vi "Task Messung.vi"(3 "Gauge":refnum<vi>, 5 "Chart":refnum<vi>, 6 "Average":refnum<vi>, 7 "Graph":refnum<vi>, 11 "Channel in":T1) -> (0 "error out":errorcluster)   [LabVIEW 2018]
uses:
  <extravilib>/ChannelInstances/Tag-t'States Worker.ctl'/))Channel.ctl
  Type Definitions/States Worker.ctl
  <vilib>/DAQmx/read.llb/DAQmx Read (Analog Wfm 1Chan NSamp).vi
  <extravilib>/ChannelInstances/Tag-t'States Worker.ctl'/Read With Abort.vi
  <extravilib>/ChannelInstances/Tag-t'States Worker.ctl'/EndpointRead.vi
  <vilib>/DAQmx/miscellaneous.llb/DAQmx Fill In Error Info.vi
  <vilib>/Waveform/WDTOps.llb/WDT Append Waveforms DBL.vi
  <extravilib>/ChannelInstances/Tag-t'States Worker.ctl'.lvlib
panel:
  out "Number of Scans":i32
  # "Worker Task"
  # "Tasks:\n1) Messen\n2) Auswerten\n3) Pausieren"
  # "Communication:\nTag Channel"
  # "These tasks run in parallel\nto other loops!"
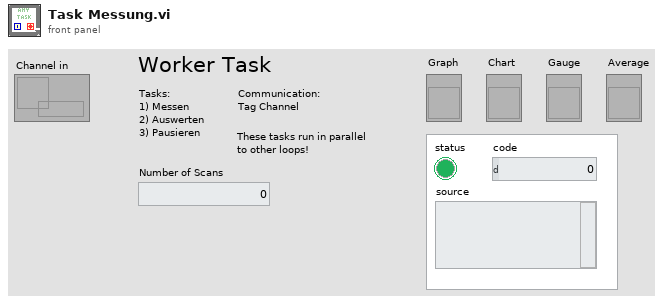
[diagram p1: front panel]
types:
  T1 = typedef "Tag-t'States Worker.ctl'.lvlib/))Channel.ctl" = refnum<queue>
  T2 = typedef "States Worker.ctl" = enum16{"Messen", "Pausieren", "Exit"}
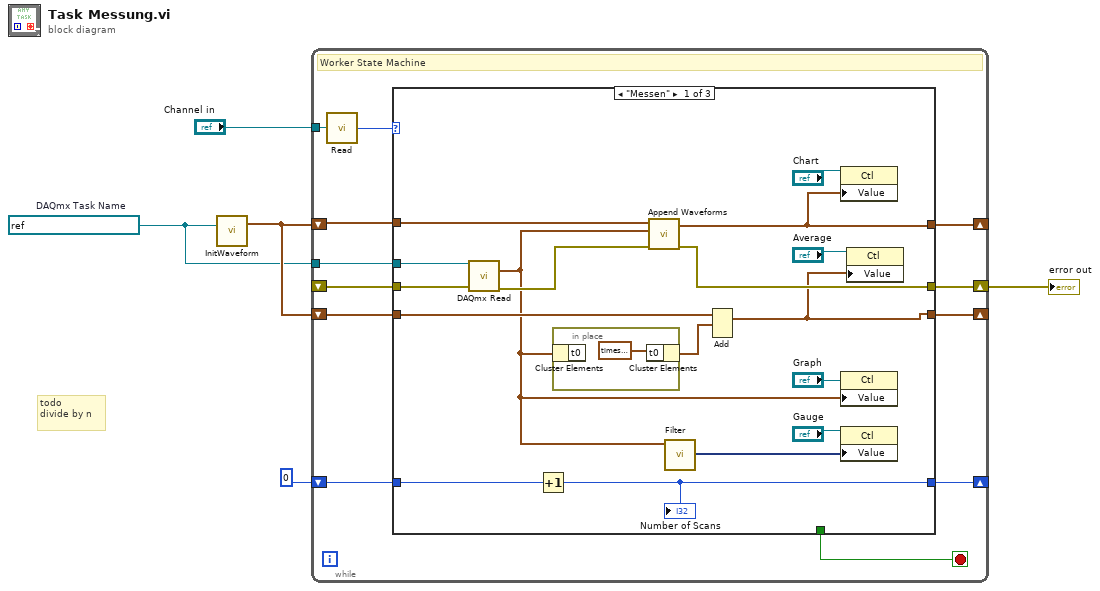
[diagram p0: block diagram]
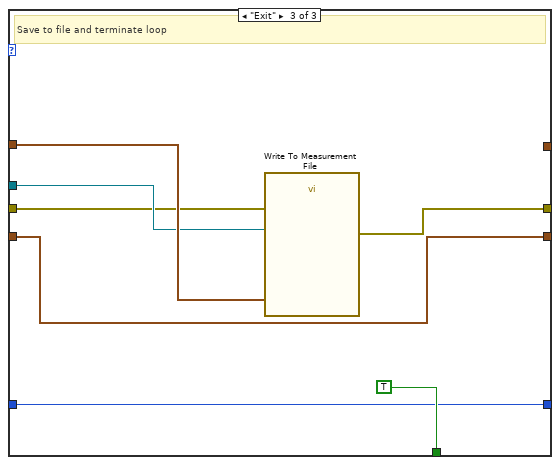
[diagram p3: hidden frame]
diagram:
  w2 = refnum<k21> "Spannung_1kHz100"  # DAQmx Task Name
  # "todo\ndivide by n"
  n1 = call "InitWaveform.vi"("Refnum in"=w2) -> ("Waveform"=w3:waveform(dbl))  [unwired: 10 in]
  n2 = while {
    shift-right: [w17] -> w5
    shift-left: _ -> [w16]
    tunnel: w2 -> [w15]
    shift-right: [w13] -> _
    shift-left: w3 -> [w14]
    shift-right: [w10] -> _
    shift-left: w3 -> [w11]
    tunnel: "Channel in" -> [w9]
    shift-right: [w6] -> _
    shift-left: 0 -> [w7]
    stop <- w12 stop-if-true
    # "Worker State Machine"
    n3 = call <extravilib>:"Read.vi"("channel"=w9) -> ("element"=w8:T2)  [unwired: 1 in, 1 out]
    n4 = case shown="\"Messen\"" w8 {
      tunnel: [w31 w38 w42] -> w17
      tunnel: w16 -> [w34 w38 w43]
      tunnel: w15 -> [w33 _ w44]
      tunnel: w14 -> [w25 w39 w45]
      tunnel: [w30 w39 _] -> w13
      tunnel: [_ _ TRUE ("abort")] -> w12
      tunnel: w11 -> [w24 w37 w41]
      tunnel: [w18 w37 w41] -> w10
      tunnel: w7 -> [w21 w36 w40]
      tunnel: [w19 w36 w40] -> w6
      frame "Messen" {
        n5 = call-poly <vilib>:"DAQmx Read.vi"("task/channels in"=w33, "error in"=w34) -> ("data"=w23:waveform(dbl), "error out"=w32:errorcluster)  [unwired: 11 in, 1 out]
        n6 = Increment(x=w21) -> (x+1=w19:i32)
        "Number of Scans" <- w19
        n7 = in-place "In Place Element Structure" {
          n8 = in-place-cluster #1(w23) -> ()  [unwired: 1 out]
          n9 = in-place-cluster #1("t0"=timestamp(0 s since 1904-01-01)) -> (w22:waveform(dbl))
        }
        n10 = call-poly <vilib>:"Append Waveforms.vi"("error in (no error)"=w32, "waveform B"=w23, "waveform A"=w25) -> ("error out"=w31:errorcluster, "waveform out"=w30:waveform(dbl))  [unwired: 7 in]
        n11 = call "Filter"("Signal"=w23) -> ("Filtered Signal"=w27:dynamicdata)  [unwired: 9 in, 1 out]
        n12 = Add(1:w22, 2:w24) -> (0:w18:waveform(dbl))  [unwired: 1 in, 1 out]
        n13 = property class="Ctl"(reference="Chart", "Value"=w30) -> ()  [unwired: 1 in, 2 out]
        n14 = property class="Ctl"(reference="Graph", "Value"=w23) -> ()  [unwired: 1 in, 2 out]
        n15 = property class="Ctl"(reference="Gauge", "Value"=w27) -> ()  [unwired: 1 in, 2 out]
        n16 = property class="Ctl"(reference="Average", "Value"=w18) -> ()  [unwired: 1 in, 2 out]
      }
      frame "Pausieren" {
        # "Do nothing, wait"
      }
      frame "Exit" {
        # "Save to file and terminate loop"
        n17 = call "Write To Measurement File"("Signals"=w45, "error in (no error)"=w43, "DAQmx Task"=w44) -> ("error out"=w42:errorcluster)  [unwired: 14 in, 2 out]
      }
    }
  }
  "error out" <- w5
